vi "Ready to Release.vi"(8 "error in (no error)":errorcluster, 11 "CubeLogger in":refnum<class "CubeLogger.lvclass">) -> (0 "error out":errorcluster, 2 "Ready to Release?":bool, 3 "CubeLogger out":refnum<class "CubeLogger.lvclass">)   [LabVIEW 2018, in "CubeLogger.lvclass"]
uses:
  CubeLogger.lvclass
  CubeLogger.lvclass/CubeLogger.ctl
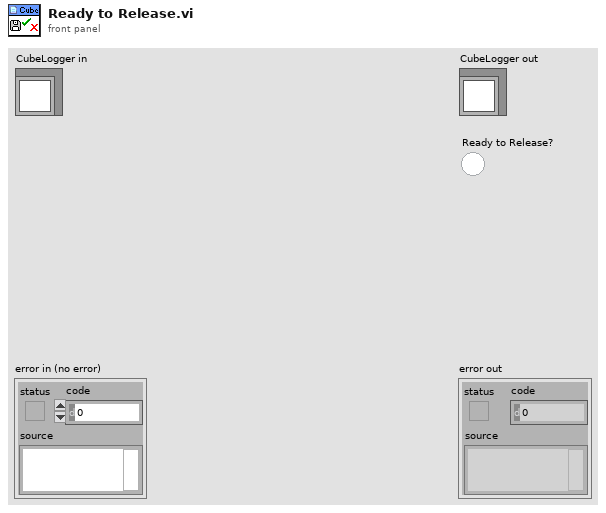
[diagram p1: front panel]
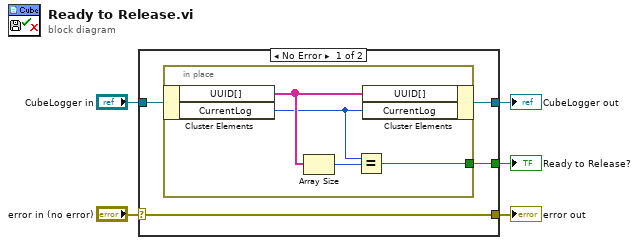
[diagram p0: block diagram]
diagram:
  n1 = case shown="No Error" "error in (no error)" {
    selector: "error in (no error)" -> [w9 w15]
    tunnel: [w9 w15] -> w4
    tunnel: [w7 w14] -> w2
    tunnel: "CubeLogger in" -> [w8 w14]
    tunnel: [w6 _] -> w1
    frame No Error {
      n2 = in-place {
        in-place-border: [w10] -> w6
        n3 = in-place-cluster #1(w8) -> ("UUID[]"=w13:string[], "CurrentLog"=w11:i32)
        n4 = Array Size(array=w13) -> (size(s)=w12:i32)
        n5 = Equal?(x=w11, y=w12) -> (x = y?=w10:bool)
        n6 = in-place-cluster #1("UUID[]"=w13, "CurrentLog"=w11) -> (w7:refnum<class "CubeLogger.lvclass">)
      }
    }
    frame Error {
    }
  }
  "error out" <- w4
  "CubeLogger out" <- w2
  "Ready to Release?" <- w1
